vi "exnFormulaConfig formula scratch pad.vi"() -> ()   [LabVIEW 2020]
panel:
  out "output variable":dbl
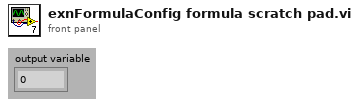
[diagram p1: front panel]
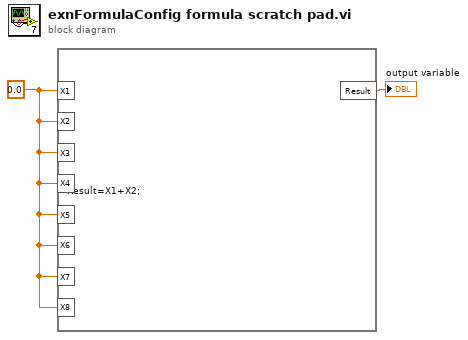
[diagram p0: block diagram]
diagram:
  w1 = 0.0 ("input variable")
  n1 = formula code="Result=X1+X2;"("X1"=w1, "X2"=w1, "X3"=w1, "X4"=w1, "X5"=w1, "X6"=w1, "X7"=w1, "X8"=w1) -> ("Result"=→"output variable":dbl)
